vi "Fehler Zaehler.vi"(6 "Aktionen":T1) -> (0 "Fehlerzähler":string, 1 "Fehlerzähler":u16, 2 "Fehler Nummern":string, 3 "Fehler Nummern":i32[](array[numeric]))   [LabVIEW 2020, in "AK-Schnittstelle.lvlib"]
uses:
  AK-Schnittstelle.lvlib
  Aktionen Stoernummern pruefen.ctl
  Stoerungen/FGV Stoermeldungen Aktion.ctl
  Stoerungen/Stoerungen.lvlib
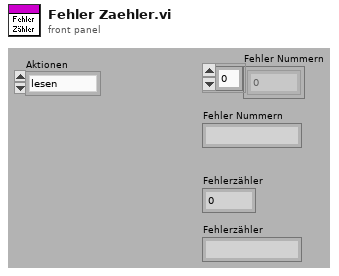
[diagram p1: front panel]
types:
  T1 = typedef "AK-Schnittstelle.lvlib/Aktionen Stoernummern pruefen.ctl" = enum16{"lesen", "prüfen"}
  T2 = typedef "Stoerungen.lvlib/FGV Stoermeldungen Aktion.ctl" = enum16{"Initialisieren", "kommend", "gehend", "lesen", "Queue leeren", "Queue freigeben", "in Datei loggen", "Änderung zurücksetzen"}
  T3 = typedef "Stoerungen.lvlib/Stoermeldung.ctl" = cluster{"Zeitstempel":timestamp, "Nummer":i32, "Kommend":bool}
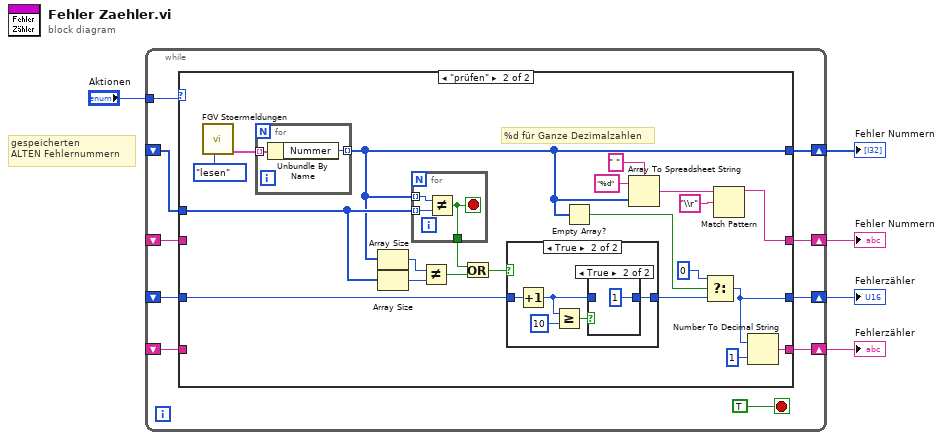
[diagram p0: block diagram]
diagram:
  # "gespeicherten\nALTEN Fehlernummern"
  n1 = while {
    shift-right: [w14] -> w4
    shift-left: _ -> [w6]
    tunnel: "Aktionen" -> [w13]
    shift-right: [w12] -> w3
    shift-left: _ -> [w11]
    shift-right: [w10] -> w2
    shift-left: _ -> [w7]
    shift-right: [w9] -> w1
    shift-left: _ -> [w8]
    stop <- TRUE stop-if-true
    n2 = case shown="\"prüfen\"" w13 {
      tunnel: w6 -> [w19 w26]
      tunnel: [w19 w25] -> w14
      tunnel: [w18 w29] -> w12
      tunnel: w11 -> [w18 w40]
      tunnel: [w16 w39] -> w10
      tunnel: [w17 w34] -> w9
      tunnel: w8 -> [w17 _]
      tunnel: w7 -> [w16 _]
      frame "lesen", Default {
      }
      frame "prüfen" {
        # "%d für Ganze Dezimalzahlen"
        n3 = call "FGV Stoermeldungen.vi"("Aktion"=FGV_Stoermeldungen_Aktion."lesen") -> ("Anzeige Array"=w31:T3[])  [unwired: 3 in, 7 out]
        n4 = for {
          tunnel: w31 -> [w45] mode=indexing
          tunnel: [w44] -> w25 mode=indexing
          n5 = Unbundle By Name(w45) -> ("Nummer"=w44:i32)
        }
        n6 = Array Size(array=w25) -> (size(s)=w22:i32)
        n7 = Array Size(array=w26) -> (size(s)=w21:i32)
        n8 = for {
          tunnel: w26 -> [w42] mode=indexing
          tunnel: w25 -> [w43] mode=indexing
          tunnel: [w41] -> w24
          stop <- w41 stop-if-true
          n9 = Not Equal?(x=w43, y=w42) -> (x != y?=w41:bool)
        }
        n10 = Not Equal?(x=w22, y=w21) -> (x != y?=w23:bool)
        n11 = Or(x=w24, y=w23) -> (x .or. y?=w20:bool)
        n12 = case shown="True" w20 {
          tunnel: w40 -> [w46 w51]
          tunnel: [w46 w47] -> w28
          frame False {
          }
          frame True {
            n13 = Increment(x=w51) -> (x+1=w48:u16)
            n14 = Greater Or Equal?(x=w48, y=u16 10) -> (x >= y?=w49:bool)
            n15 = case shown="True" w49 {
              tunnel: w48 -> [w52 _]
              tunnel: [w52 u16 1 ("y")] -> w47
              frame False {
              }
              frame True {
              }
            }
          }
        }
        n16 = Empty Array?(array=w25) -> (empty?=w27:bool)
        n17 = Array To Spreadsheet String(delimiter (Tab)=" " ("Trennzeichen (Tabulator)"), array=w25, 3:"%d" ("Format-String")) -> (spreadsheet string=w35:string)
        n18 = Select(t=u16 0, s=w27, f=w28) -> (s? t:f=w29:u16)
        n19 = Match Pattern(string=w35, regular expression="\\r" ("Nach String/Zeichen suchen (-)")) -> (before substring=w34:string)  [unwired: 1 in, 3 out]
        n20 = Number To Decimal String(number=w29, width (-)=i16 1 ("Breite (-)")) -> (decimal integer string=w39:string)
      }
    }
  }
  "Fehler Nummern" <- w4
  "Fehlerzähler" <- w3
  "Fehlerzähler" <- w2
  "Fehler Nummern" <- w1
